vi "TEST.vi"(8 "Array":dbl[](array[numeric])=[0.12345678901234568, 1.1234567890123457, 2.1234567890123457, 3.1234567890123457, 4.123456789012345, 5.123456789012345] format="%_30f") -> (0 "Array 2":dbl[](array[numeric]) format="%_30f", 4 "Zahl":dbl[](array[numeric]) format="%_18f", 6 "String in F-Format":string[](array[string]))   [LabVIEW 2020, in "Linearisierung v2.lvlib"]
uses:
  Linearisierung v2.lvlib
  Visualisierungs Elemente/String - Ausgabefeld.ctl
  Visualisierungs Elemente/Auswahlfeld.ctl
  Seiten/FT-IR/FGV FT-IR Gasliste Aktionen.ctl
  Seiten/System Einstellungen V2/Gasflaschenkomponente.ctl
  PDF_Interface/PDF Protokoll Standard Kopf Optionen.ctl
  Aktion Lin Daten aufarbeiten.ctl
  SpanEinstellungen/Aktion FGV SpanEinstellungen.ctl
  Seiten/System Einstellungen V2/Konfig Gasflasche.ctl
  <vilib>/regexp/Match Regular Expression.xnode
  Seiten/System Einstellungen V2/System Einstellungen V2.lvlib
  Seiten/FT-IR/FT-IR.lvlib
  Protokoll/Protokoll.lvlib
  PDF_Interface/PDF Interface.lvlib
  Gasteiler/Gasteiler.lvlib
  SpanEinstellungen/SpanEinstellungen.lvlib
panel:
  in  "Array 7":void[](array[numeric])
  out "Numerisches Anzeigeelement":dbl[](array[numeric])
  out "NXG Numerisches Anzeigeelement":dbl[](array[numeric])
  out "Numerisch Standard":dbl[](array[numeric])
  out "Numerisches Element":dbl[](array[numeric])
  out "MFC Flow Cluster":cluster{"min flow":dbl, "max flow":dbl}[](array[cluster]) caption="MFC Flow"
  out "Array 5":string[][][](array[string])
  in  "Einheiten":string[](array[string])
  out "Array 6":string[](array[string])
  out "Teil-Array":string[][](array[string])
  out "Stufentabellen":string[][][](array[string])
  out "Stufen ja Gas":string[][](array[string])
  in  "Gas Namen":string[](array[string])=["O2", "CO2", "Xe"]
  out "Array 4":string[](array[string])
  out "Array 3":string[](array[string])
  in  "Empfangsdaten":string[](array[string])=["CO2", "1.729", "N2", "9.83", "O2", "1.642", "Xe", "8.643"]
  out "Angehängtes Array":i32[](array[numeric])
  out "Offset nach Übereinstimmung 2":i32
  out "Header Labels":string[](array[string])
  out "Header Values":T1[](array[typedef])
  out "Aktuelle Gasliste gesamt":T1[](array[typedef])
  out "Autorange Bereiche 2":T2[](array[typedef])
  out "Autorange Bereiche":T1[](array[typedef])
  out "Offset nach Übereinstimmung":i32
  out "Übereinstimmender Teil-String":string
  in  "Komp":string
  out "Konzentration IST":dbl
  out "Gasauswahl":string
  out "found":bool[](array[boolean])
  out "Konzentrationen":dbl[](array[numeric])
  out "Gasliste":string[](array[string])
  out "Channel found":bool
  out "Konzentration out":dbl
  in  "Komponente":string
  out "x*y":dbl
  out "x+y":dbl
  # "CO2 1.729\nN2 9.983E+08\nNO2 1.729\nO2 1.642E+06\nXe 8.643E+04"
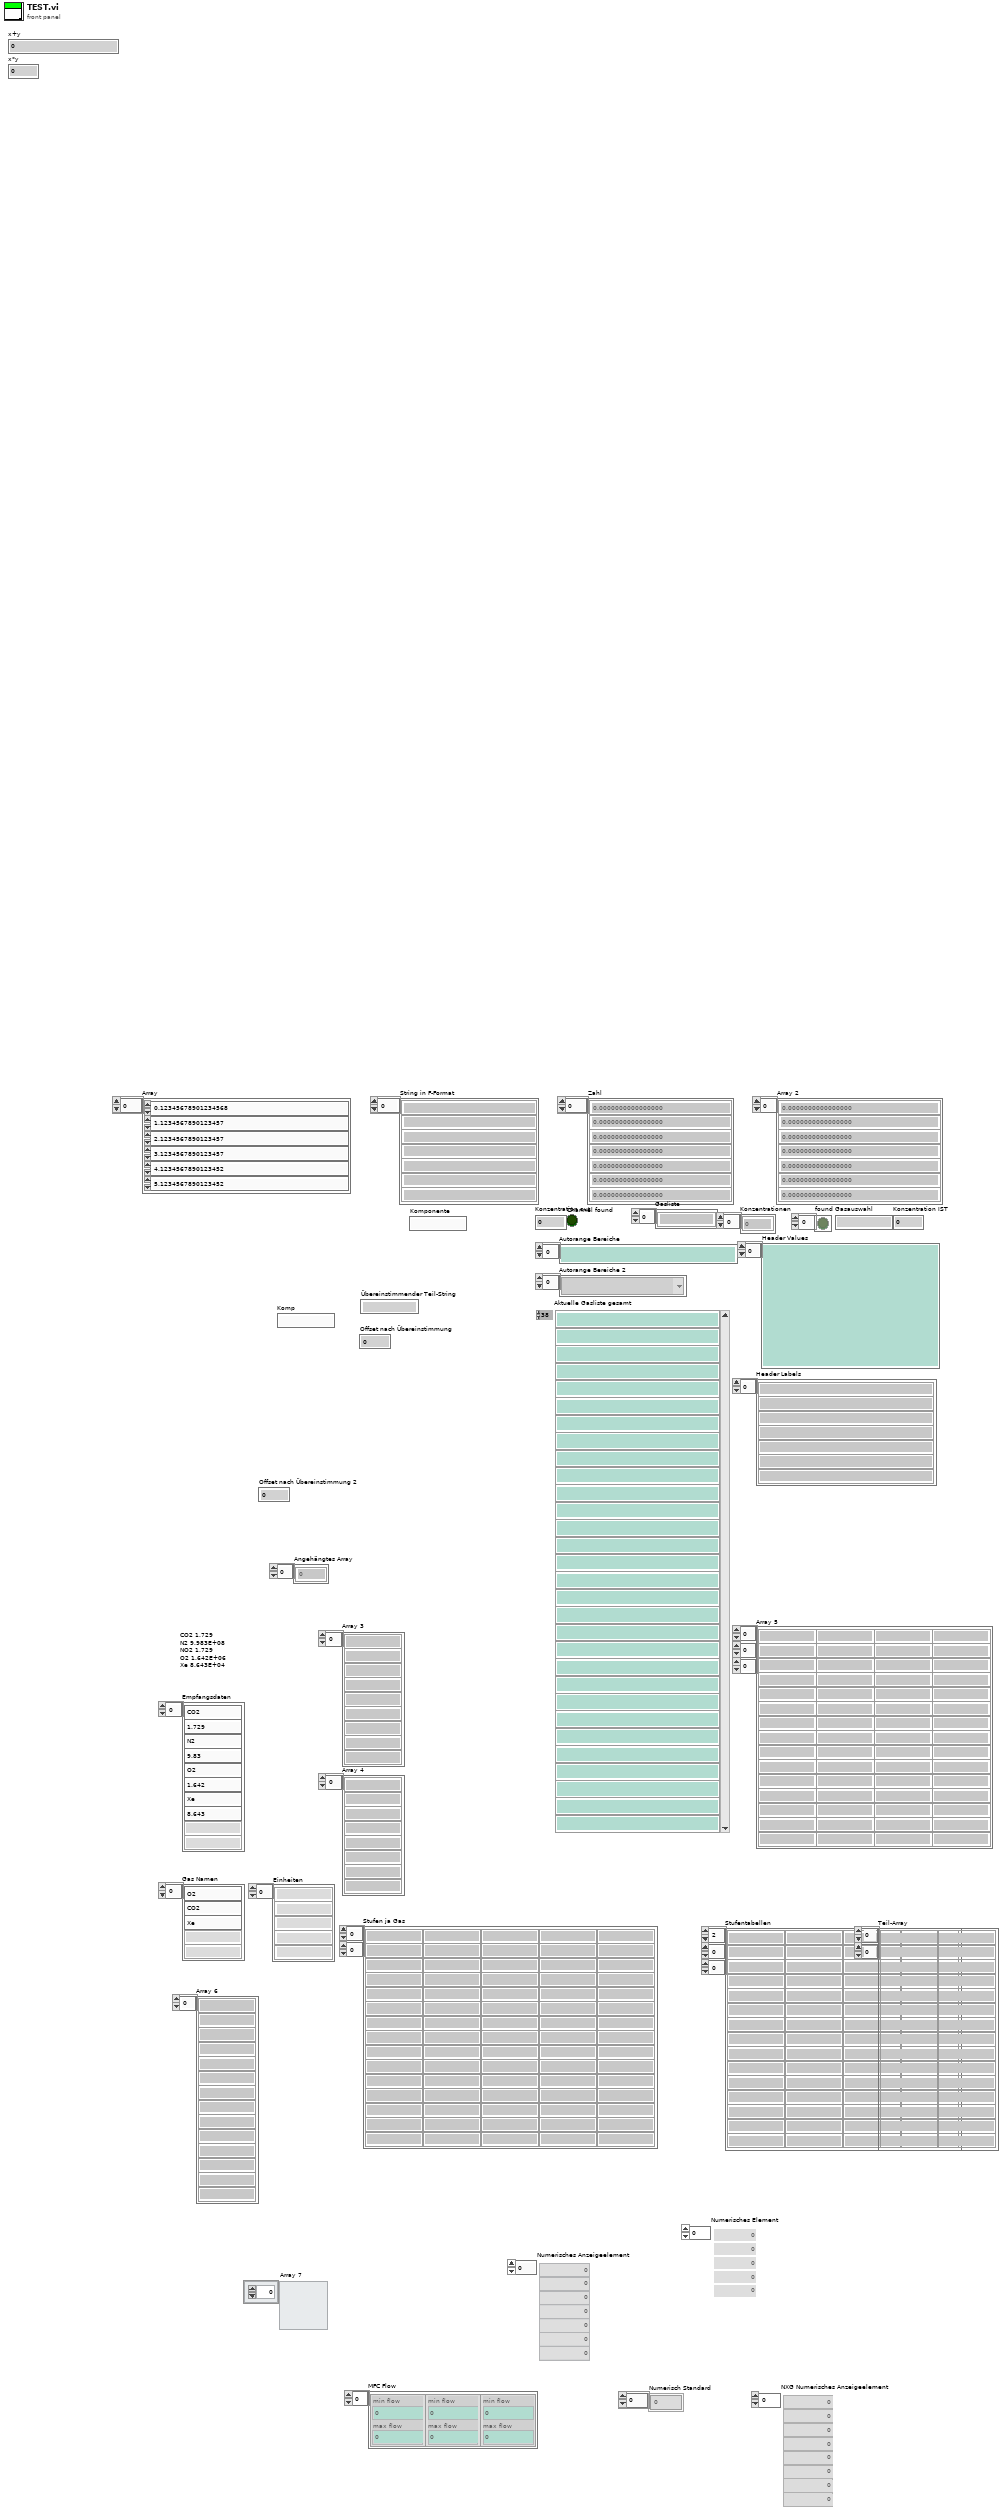
[diagram p1: front panel]
types:
  T1 = typedef "String - Ausgabefeld.ctl" = string
  T2 = typedef "Auswahlfeld.ctl" = u16
  T3 = typedef "System Einstellungen V2.lvlib/Konfig Gasflasche.ctl" = bool
  T4 = typedef "Linearisierung v2.lvlib/SpanEinstellungen.lvlib/Aktion FGV SpanEinstellungen.ctl" = enum16{"lesen", "schreiben", "laden", "speichern", "RegisterRef", "automatisch", "init", "PDF Params", "Punkte umkehren"}
  T5 = typedef "Linearisierung v2.lvlib/Aktion Lin Daten aufarbeiten.ctl" = enum16{"lesen", "Protkolldaten", "speichern", "laden", "EPA auswerten", "Tabelle schreiben", "Lin auswerten", "Tab init", "Stufentabelle", "EPA aktiviert", "Nachbehandlung laden", "Tabelle löschen", "Istwerte löschen", "Zeile löschen", "Zeile einfügen", "LIN aktiviert", "LIN/EPA aktiv laden", "EGAK Tab", "LIN übernehmen"}
  T6 = typedef "PDF Interface.lvlib/PDF Protokoll Standard Kopf Optionen.ctl" = cluster{"Analysator":bool, "FT-IR Rezept":bool, "Gasteiler":bool, "Gas Komponente":bool, "Gas Flasche":bool, "LIN Protokoll":bool, "Operator":bool}
  T7 = typedef "FT-IR.lvlib/FGV FT-IR Gasliste Aktionen.ctl" = enum16{"lesen", "Gasliste FT-IR", "Gasliste ausgelesen", "laden", "speichern", "löschen"}
  T8 = typedef "System Einstellungen V2.lvlib/Gasflaschenkomponente.ctl" = cluster{"Gasauswahl":string, "Konzentration IST":dbl, "Einheit":string, "Genauigkeit":dbl}
  T9 = typedef "Linearisierung v2.lvlib/SpanEinstellungen.lvlib/SpanInletCluster.ctl" = cluster{"Span Inlet Active":T3, "Analysator":T10, "Konfig Gasflasche":T3, "Gasflasche":T11, "Gasflaschen Nr.:":string, "Ablaufdatum":timestamp, "Komponenten":T12, "Zeitdauer Stufen":sgl, "Max Fehler":sgl, "Anzahl Stufen":sgl, "Trägergas":T16, "zusätzliche Zeitdauer Erster Punkt":sgl}
  T10 = typedef "System Einstellungen V2.lvlib/Analysatoren.ctl" = string
  T11 = typedef "System Einstellungen V2.lvlib/Gasflasche Auswahl.ctl" = u16
  T12 = typedef "Linearisierung v2.lvlib/SpanEinstellungen.lvlib/Komponentencluster mit Formel.ctl" = cluster{"Komponente 1":T13, "Komponente 2":T13, "Komponente 3":T13, "Komponente 4":T13, "Komponente 5":T13}
  T13 = typedef "Linearisierung v2.lvlib/SpanEinstellungen.lvlib/Komponentenauswahl mit Formel.ctl" = cluster{"Komponente:":u16, "Summenformel":T14, "Konzentration IST":dbl, "Einheit":T15, "Genauigkeit":dbl}
  T14 = typedef "String - Eingabefeld.ctl" = string
  T15 = typedef "Linearisierung v2.lvlib/SpanEinstellungen.lvlib/Einheit.ctl" = enum16{"ppm", "%"}
  T16 = typedef "System Einstellungen V2.lvlib/Traegergas.ctl" = string
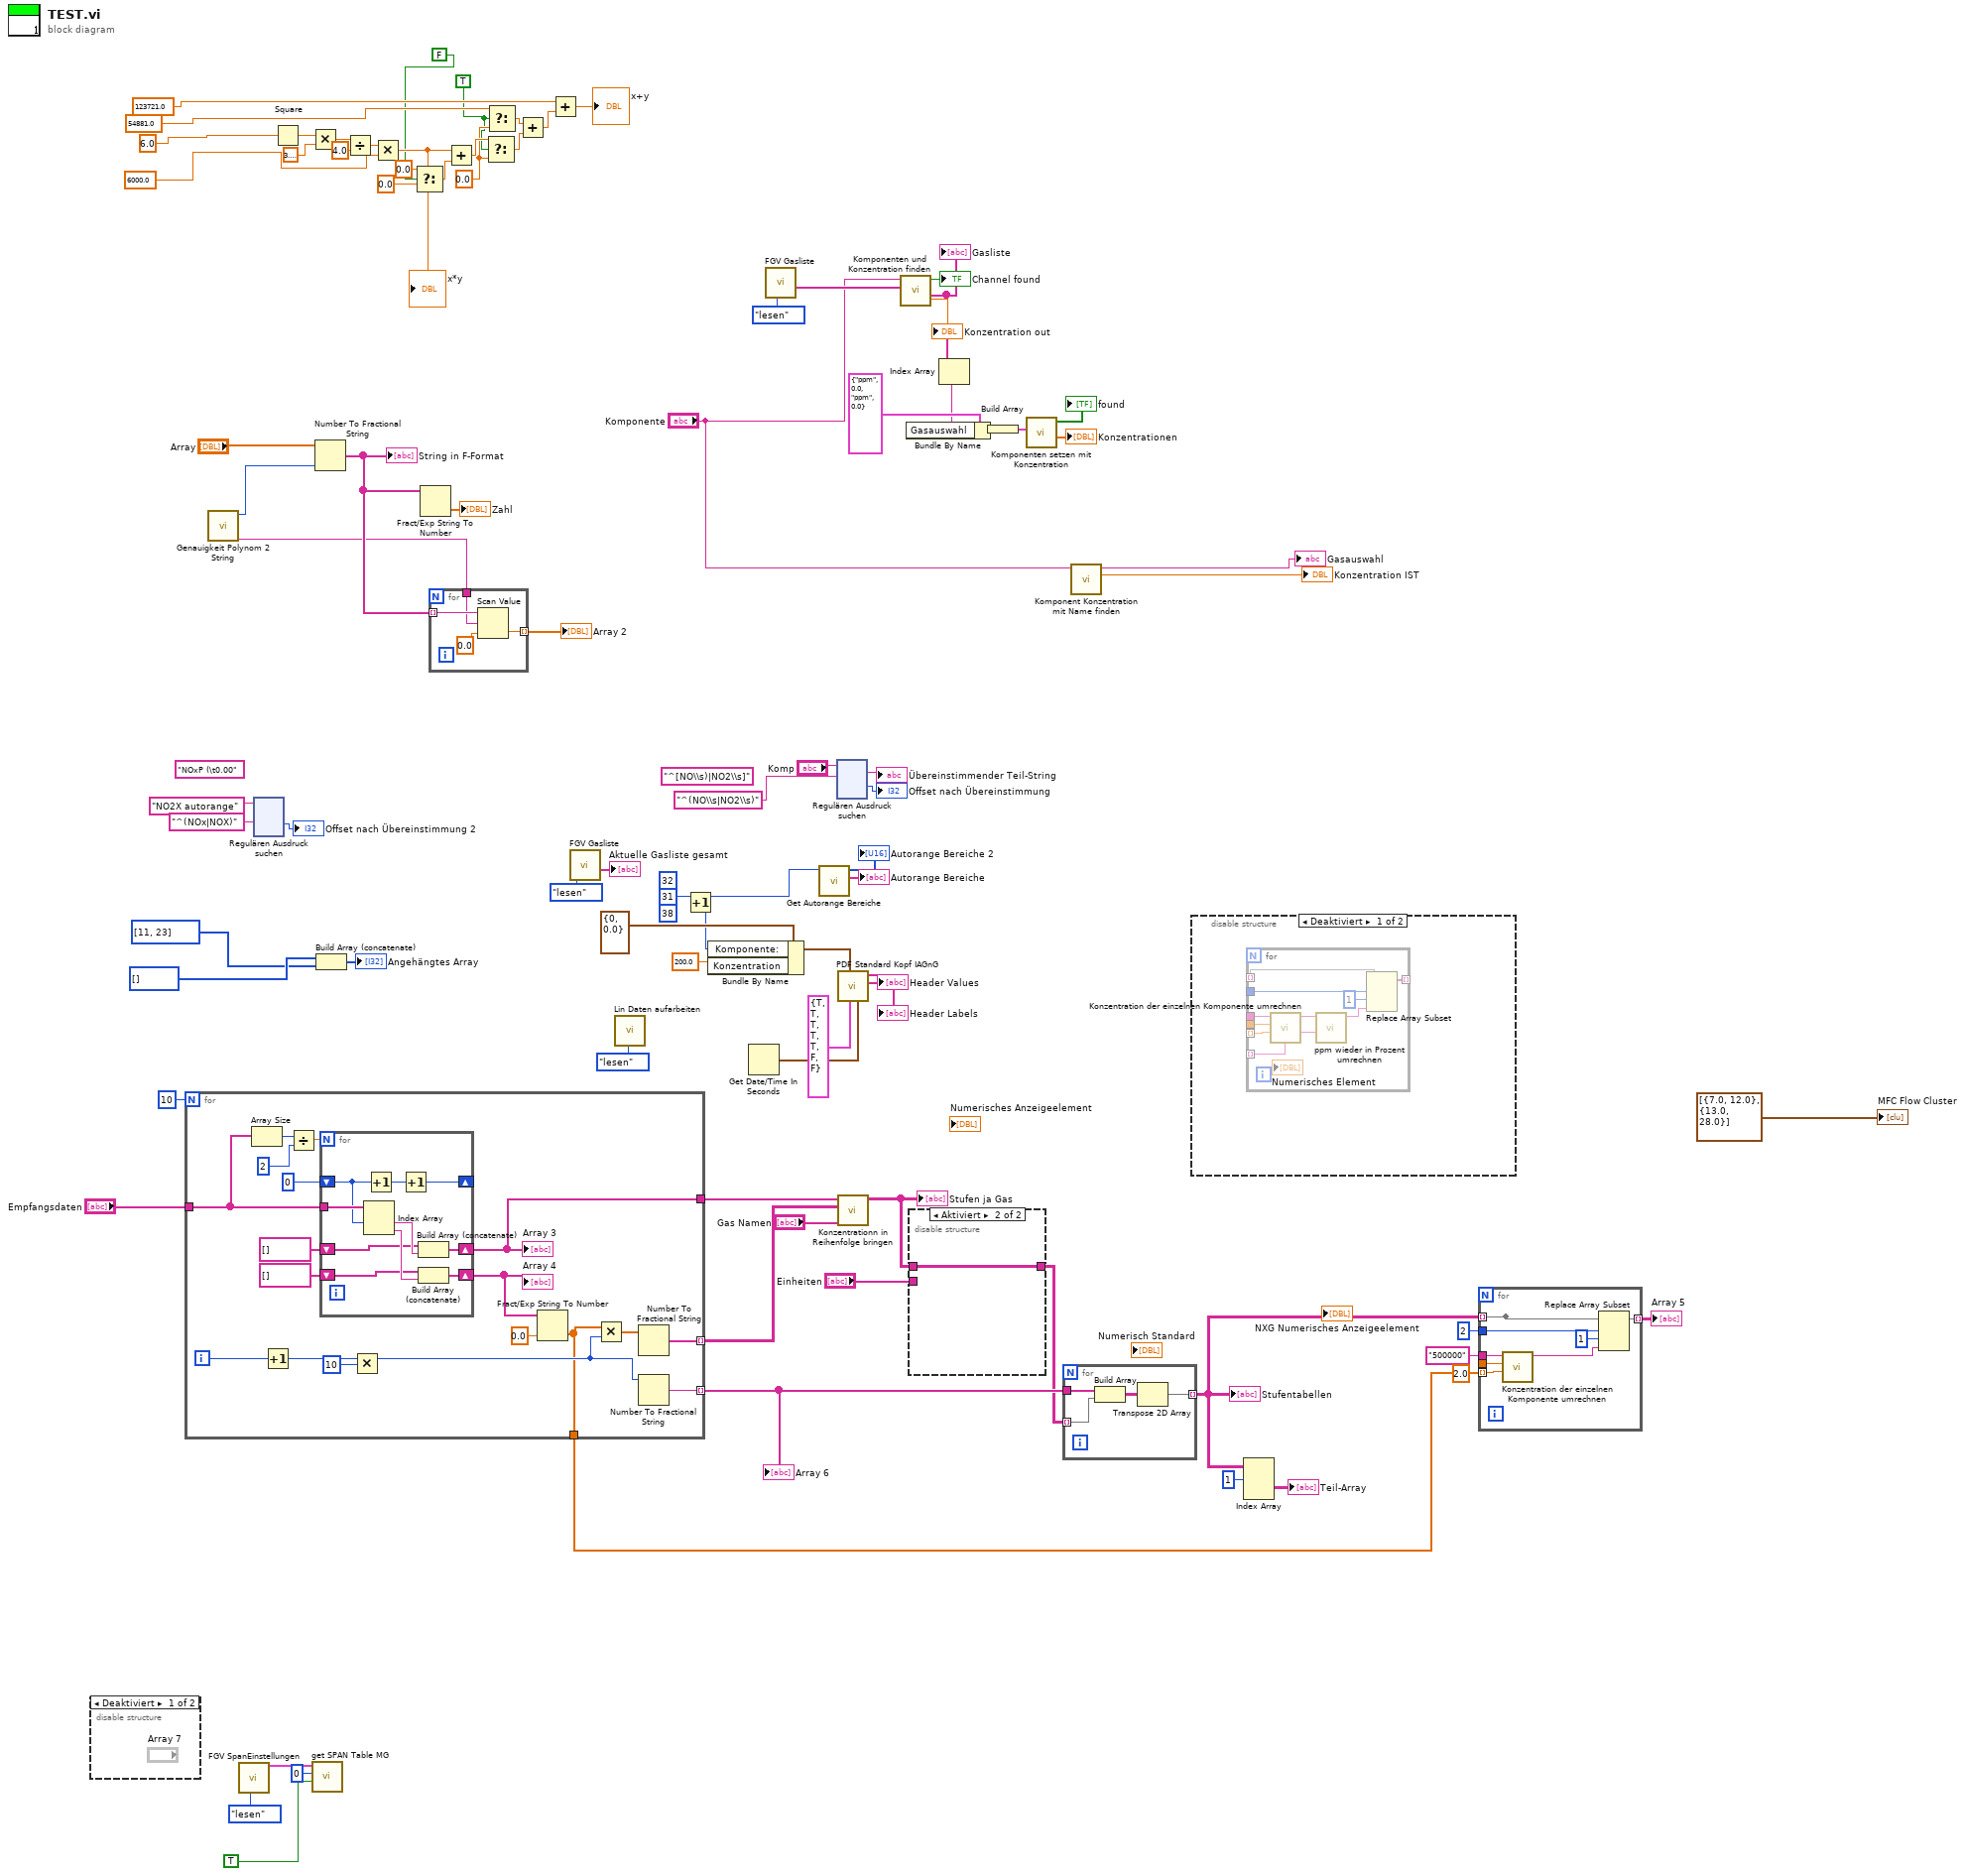
[diagram p0: block diagram]
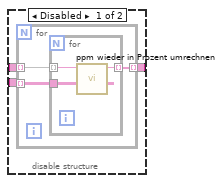
[diagram p4: hidden frame]
diagram:
  (unwired) "NOxP (\t0.00" ("String")
  (unwired) 38
  w31 = 31
  (unwired) 32
  (unwired) "^[NO\\s)|NO2\\s]" ("t")
  w71 = TRUE
  w75 = sgl 0.0 ("f")
  n1 = disable-structure shown="Deaktiviert" {
    frame Disabled {
    }
    frame Enabled {
    }
  }
  n2 = for {
    N: 10 -> [_]
    tunnel: "Empfangsdaten" -> [w103]
    tunnel: [w95] -> w19 mode=indexing
    tunnel: [w94] -> w20
    tunnel: [w89] -> w15 mode=indexing
    tunnel: [w88] -> w8
    i -> [w92]
    n3 = Array Size(array=w103) -> (size(s)=w102:i32)
    n4 = Increment(x=w92) -> (x+1=w91:i32)
    n5 = Divide(x=w102, y=2) -> (x/y=w100:dbl)
    n6 = for {
      N: w100 -> [_]
      shift-right: [w113] -> w94
      shift-left: string[] [] -> [w111]
      shift-right: [w112] -> w98
      shift-left: string[] [] -> [w110]
      tunnel: w103 -> [w109]
      shift-right: [w106] -> _
      shift-left: 0 ("y") -> [w108]
      n7 = Index Array(array=w109, index #1=w108) -> (element #1=w115:string, element #2=w114:string)  [unwired: 1 in]
      n8 = Increment(x=w108) -> (x+1=w107:i32)
      n9 = Increment(x=w107) -> (x+1=w106:i32)
      n10 = Build Array (concatenate)(w111, w115) -> (w113:string[])
      n11 = Build Array (concatenate)(w110, w114) -> (w112:string[])
    }
    "Array 3" <- w94
    "Array 4" <- w98
    n12 = Multiply(x=w91, y=10) -> (x*y=w90:i32)
    n13 = Fract/Exp String To Number(string=w98, default (0 dbl)=0.0 ("Standard (0 DBL)")) -> (number=w88:dbl[])  [unwired: 2 in, 1 out]
    n14 = Multiply(x=w88, y=w90) -> (x*y=w96:dbl[])
    n15 = Number To Fractional String(number=w96) -> (F-format string=w95:string[])  [unwired: 3 in]
    n16 = Number To Fractional String(number=w90) -> (F-format string=w89:string)  [unwired: 3 in]
  }
  "Array 6" <- w15
  n17 = call "Genauigkeit Polynom 2 String.vi"() -> ("Format-String Polynom 2 Sting"=w62:string, "Genauigkeit Polynom 2 String"=w63:i16)  [unwired: 9 in, 1 out]
  n18 = call "FGV SpanEinstellungen.vi"("Aktion"=Aktion_FGV_SpanEinstellungen."lesen") -> ("SpanInletClusterArray out"=w3:T9[])  [unwired: 6 in, 4 out]
  n19 = xnode "Regulären Ausdruck suchen"("Eingangs-String"="NO2X autorange" ("String"), "Regulärer Ausdruck"="^(NOx|NOX)") -> ("Offset nach Übereinstimmung"=→"Offset nach Übereinstimmung 2":i32)  [unwired: 4 in, 4 out]
  n20 = Square(x=6.0) -> (x^2=w87:dbl)
  n21 = Multiply(x=w87, y=sgl 3.1415927) -> (x*y=w86:dbl)
  n22 = call "get SPAN Table MG.vi"("automatisch in"=T3 TRUE, "active reprocessing SPAN"=0, "SpanInletClusterArray in"=w3) -> ()  [unwired: 2 in, 7 out]
  n23 = Number To Fractional String(number="Array", precision (6)=w63) -> (F-format string=w64:string[])  [unwired: 2 in]
  "String in F-Format" <- w64
  n24 = Build Array (concatenate)(i32[] [], i32[] [11, 23]) -> (→"Angehängtes Array":i32[])
  n25 = Divide(x=w86, y=sgl 4.0) -> (x/y=w84:dbl)
  n26 = Multiply(x=w84, y=6000.0 ("x")) -> (x*y=w83:dbl)
  "x*y" <- w83
  n27 = Select(t=sgl 0.0, s=FALSE, f=sgl 0.0) -> (s? t:f=w79:sgl)
  n28 = Fract/Exp String To Number(string=w64) -> (number=→"Zahl":dbl[])  [unwired: 3 in, 1 out]
  n29 = for {
    tunnel: w64 -> [w119] mode=indexing
    tunnel: [w118] -> w61 mode=indexing
    tunnel: w62 -> [w116]
    n30 = Scan Value(string=w119, format string=w116, default (0 dbl)=0.0) -> (value=w118:dbl)  [unwired: 1 out]
  }
  "Array 2" <- w61
  n31 = Add(x=w83, y=w79) -> (x+y=w78:dbl)
  n32 = Select(t=w78, s=w71, f=w75) -> (s? t:f=w77:dbl)
  n33 = Select(t=sgl 54881.0 ("x"), s=w71, f=w75) -> (s? t:f=w76:sgl)
  n34 = Add(x=w76, y=w77) -> (x+y=w82:dbl)
  n35 = Add(x=sgl 123721.0, y=w82) -> (x+y=→"x+y":dbl)
  n36 = call "FGV Gasliste.vi"("Aktionen"=FGV_FT-IR_Gasliste_Aktionen."lesen") -> ("Aktuelle Gasliste gesamt"=→"Aktuelle Gasliste gesamt":T1[])  [unwired: 8 in, 2 out]
  n37 = call "Lin Daten aufarbeiten.vi"("Aktionen"=Aktion_Lin_Daten_aufarbeiten."lesen") -> ()  [unwired: 16 in, 11 out]
  n38 = Increment(x=w31) -> (x+1=w29:i32)
  n39 = Bundle By Name(cluster=cluster{"Komponente:":T2, "Konzentration":dbl} {"Komponente:"=0, "Konzentration"=0.0} ("Gas Komponente"), "Komponente:"=w29, "Konzentration"=200.0) -> (w32:cluster{"Komponente:":T2, "Konzentration":dbl})
  n40 = Get Date/Time In Seconds() -> (seconds since 1Jan1904=w35:timestamp)
  n41 = call "FGV Gasliste.vi"("Aktionen"=FGV_FT-IR_Gasliste_Aktionen."lesen") -> ("Aktuelle Gasliste gesamt"=w59:T1[])  [unwired: 8 in, 2 out]
  n42 = call "Get Autorange Bereiche.vi"("Gaskomponente"=w31) -> (2:"Autorange Bereiche"=→"Autorange Bereiche":T1[], 3:"Autorange Bereiche"=→"Autorange Bereiche 2":T2[])  [unwired: 8 in, 1 out]
  n43 = xnode "Regulären Ausdruck suchen"("Eingangs-String"="Komp", "Regulärer Ausdruck"="^(NO\\s|NO2\\s)" ("t")) -> ("Komplette Übereinstimmung"=→"Übereinstimmender Teil-String":string, "Offset nach Übereinstimmung"=→"Offset nach Übereinstimmung":i32)  [unwired: 4 in, 3 out]
  n44 = call "PDF Standard Kopf IAGnG.vi"("Zeitstempel"=w35, "Oprtionen Cluster"=T6 {"Analysator"=TRUE, "FT-IR Rezept"=TRUE, "Gasteiler"=TRUE, "Gas Komponente"=TRUE, "Gas Flasche"=TRUE, "LIN Protokoll"=FALSE, "Operator"=FALSE}, "Gas Komponente"=w32) -> ("Header Values"=→"Header Values":T1[], "Header Labels"=→"Header Labels":string[])  [unwired: 5 in, 2 out]
  n45 = call "Konzentrationn in Reihenfolge bringen.vi"("Gas Namen"="Gas Namen", "Konzentrationen"=w19, "Gase"=w20) -> ("Stufen ja Gas"=w14:string[][])  [unwired: 8 in]
  "Stufen ja Gas" <- w14
  n46 = call "Komponenten und Konzentration finden.vi"("Aktuelle Gasliste gesamt"=w59, "String"="Komponente") -> ("Gasliste"=w53:string[], "Channel found"=→"Channel found":bool, "Konzentration out"=→"Konzentration out":dbl)  [unwired: 5 in, 2 out]
  "Gasliste" <- w53
  n47 = disable-structure shown="Aktiviert" {
    disable-tunnel: w14 -> [w122 w129]
    disable-tunnel: "Einheiten" -> [w121 _]
    disable-tunnel: [w120 w129] -> w12
    frame Disabled {
      n48 = for {
        tunnel: w121 -> [w125] mode=indexing
        tunnel: w122 -> [w124] mode=indexing
        tunnel: [w123] -> w120 mode=indexing
        n49 = for {
          tunnel: w125 -> [w128]
          tunnel: w124 -> [w126] mode=indexing
          tunnel: [w127] -> w123 mode=indexing
          n50 = call "ppm wieder in Prozent umrechnen.vi"("Einheit"=w128, "Werteingang"=w126) -> ("Wertausgang"=w127:string)  [unwired: 9 in]
        }
      }
    }
    frame Enabled {
    }
  }
  n51 = Index Array(array=w53) -> (element=w52:string)  [unwired: 1 in]
  n52 = Bundle By Name(cluster=T8 {"Gasauswahl"="ppm", "Konzentration IST"=0.0, "Einheit"="ppm", "Genauigkeit"=0.0} ("Komponenten"), "Gasauswahl"=w52) -> (w55:T8)
  n53 = Build Array(w55) -> (w54:T8[])
  n54 = call "Komponenten setzen mit Konzentration.vi"("Komponenten"=w54) -> ("Konzentrationen"=→"Konzentrationen":dbl[], "found"=→"found":bool[])  [unwired: 6 in, 3 out]
  n55 = for {
    tunnel: w15 -> [w132]
    tunnel: w12 -> [w131] mode=indexing
    tunnel: [w130] -> w11 mode=indexing
    n56 = Build Array(w132, w131) -> (w133:string[][])
    n57 = Transpose 2D Array(2D array=w133) -> (transposed array=w130:string[][])
  }
  "Stufentabellen" <- w11
  n58 = call "Komponent Konzentration mit Name finden.vi"("Komponente"="Komponente") -> ("Konzentration OUT"=→"Konzentration IST":dbl, "Gasauswahl"=→"Gasauswahl":string)  [unwired: 8 in, 1 out]
  n59 = disable-structure shown="Deaktiviert" {
    frame Disabled {
      n60 = for {
        tunnel: _ -> [w141] mode=indexing
        tunnel: _ -> [w140] mode=indexing
        tunnel: _ -> [w142]
        tunnel: _ -> [w139]
        tunnel: _ -> [w136]
        tunnel: _ -> [w135] mode=indexing
        tunnel: [w134] -> _ mode=indexing
        n61 = call "Konzentration der einzelnen Komponente umrechnen.vi"("Teilkonzentration"=w141, "Gesamtkonzentration"=w139, "Werteingang"=w142) -> ("Wertausgang"=w143:string)  [unwired: 8 in]
        n62 = call "ppm wieder in Prozent umrechnen.vi"("Einheit"=w140, "Werteingang"=w143) -> ("Wertausgang"=w137:string)  [unwired: 9 in]
        n63 = Replace Array Subset(array=w135, new element=w137, index (row)=w136, index (col)=1 ("Deaktivierter Index (Spalte)")) -> (w134:string[])
      }
    }
    frame Enabled {
    }
  }
  n64 = Index Array(array=w11, index (dim 0)=1 ("Index (Seite)")) -> (element=→"Teil-Array":string[][])  [unwired: 2 in]
  n65 = for {
    tunnel: w8 -> [w150] mode=indexing
    tunnel: "500000" ("Daten (Leerstring)") -> [w151]
    tunnel: 2.0 -> [w149]
    tunnel: 2 ("Zeile") -> [w147]
    tunnel: [w145] -> _ mode=indexing
    tunnel: [w146] -> w6 mode=indexing
    tunnel: w11 -> [w145] mode=indexing
    n66 = call "Konzentration der einzelnen Komponente umrechnen.vi"("Teilkonzentration"=w150, "Gesamtkonzentration"=w149, "Werteingang"=w151) -> ("Wertausgang"=w144:string)  [unwired: 8 in]
    n67 = Replace Array Subset(array=w145, new element=w144, index (row)=w147, index (col)=1 ("Deaktivierter Index (Spalte)")) -> (w146:string[][])
  }
  "Array 5" <- w6
  "MFC Flow Cluster" <- cluster{"min flow":dbl, "max flow":dbl}[] [{"min flow"=7.0, "max flow"=12.0}, {"min flow"=13.0, "max flow"=28.0}] ("MFC Flow Cluster")
